vi "Read LSEOutput.vi"(8 "error in (no error)":errorcluster, 11 "VisualizeAppLSE in":refnum<class "VisualizeAppLSE.lvclass">) -> (0 "error out":errorcluster, 2 "LSEOutput":T1={"SystemVoltagesRef"=[], "Vestimate"=[], "LSEConfig"={"NoiseVariance"=0.001, "IEEESystem"=5, "PMULocations"=[1], "Vindex"=0, "Iindex"=3, "DynamicRef"=""}, "Bus"=[]}, 3 "VisualizeAppLSE out":refnum<class "VisualizeAppLSE.lvclass">)   [LabVIEW 2017, in "Visualization.lvlib" / "VisualizeAppLSE.lvclass"]
uses:
  VisualizeAppLSE.lvclass
  Modules/AppPlugins/LSEPlugin/PublicAPI/Typedefs/LSEOutput.ctl
  Modules/AppPlugins/LSEPlugin/PublicAPI/Typedefs/LSEConfig.ctl
  VisualizeAppLSE.lvclass/VisualizeAppLSE.ctl
  Modules/AppPlugins/LSEPlugin/LSEPlugin.lvclass
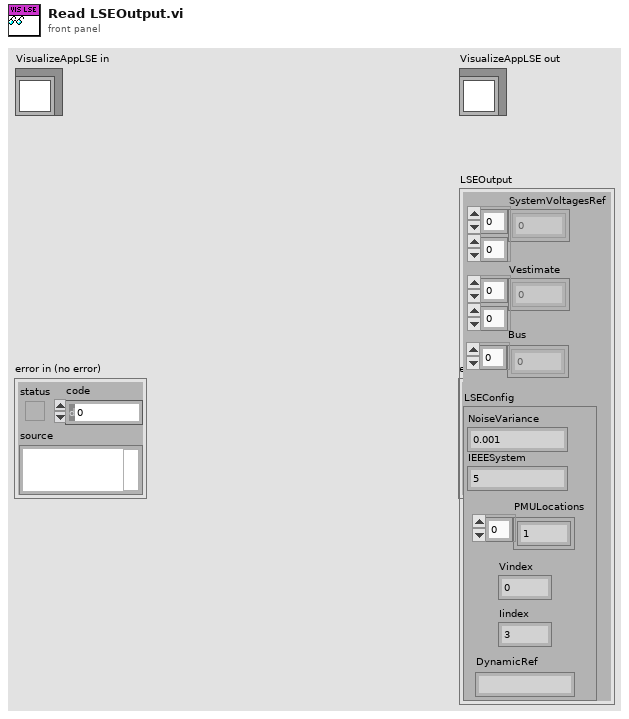
[diagram p1: front panel]
types:
  T1 = typedef "AppPlugins.lvlib/LSEPlugin.lvclass/LSEOutput.ctl" = cluster{"SystemVoltagesRef":cdb[][], "Vestimate":cdb[][], "LSEConfig":T2, "Bus":dbl[]}
  T2 = typedef "AppPlugins.lvlib/LSEPlugin.lvclass/LSEConfig.ctl" = cluster{"NoiseVariance":dbl, "IEEESystem":u32, "PMULocations":u32[], "Vindex":i32, "Iindex":i32, "DynamicRef":string}
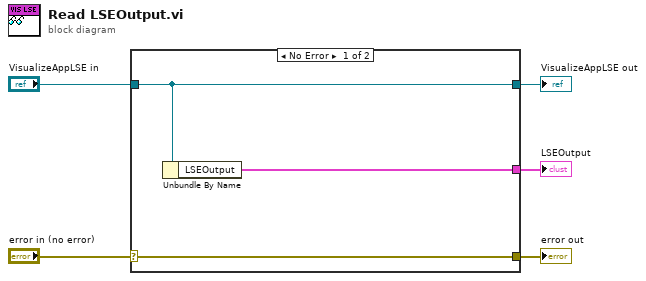
[diagram p0: block diagram]
diagram:
  n1 = case shown="No Error" "error in (no error)" {
    selector: "error in (no error)" -> [w8 w9]
    tunnel: [w8 w9] -> w4
    tunnel: [w7 w10] -> w2
    tunnel: "VisualizeAppLSE in" -> [w7 w10]
    tunnel: [w6 _] -> w1
    frame No Error {
      n2 = Unbundle By Name(w7) -> ("LSEOutput"=w6:T1)
    }
    frame Error {
    }
  }
  "error out" <- w4
  "VisualizeAppLSE out" <- w2
  "LSEOutput" <- w1
